vi "SubVI_ReadTDMs.vi"(8 "error in":errorcluster, 10 "Range Slide":cluster{dbl, dbl}={0.0, 1.0}, 11 "tdms文件输出":refnum<k34>) -> (0 "error out":errorcluster, 2 "WFM Out":waveform(dbl)[](array[waveform]), 3 "tdms file out":refnum<k34>)   [LabVIEW 2012]
panel:
  out "x*y":dbl
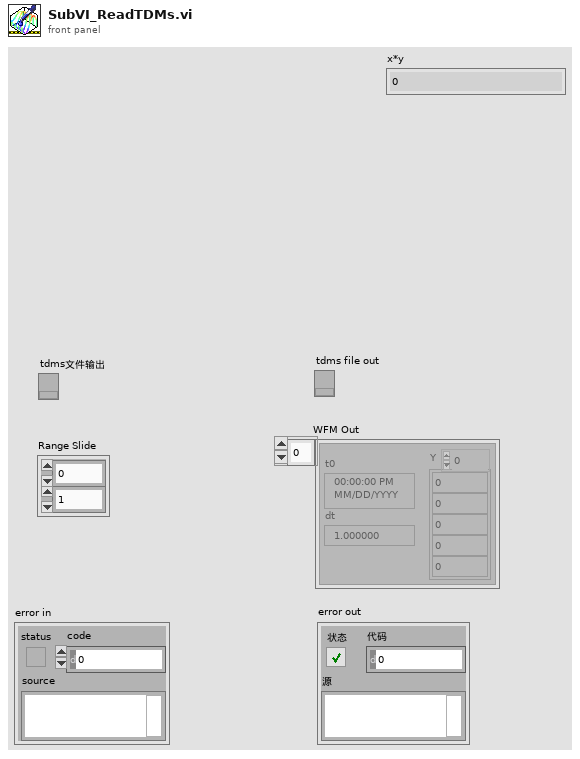
[diagram p1: front panel]
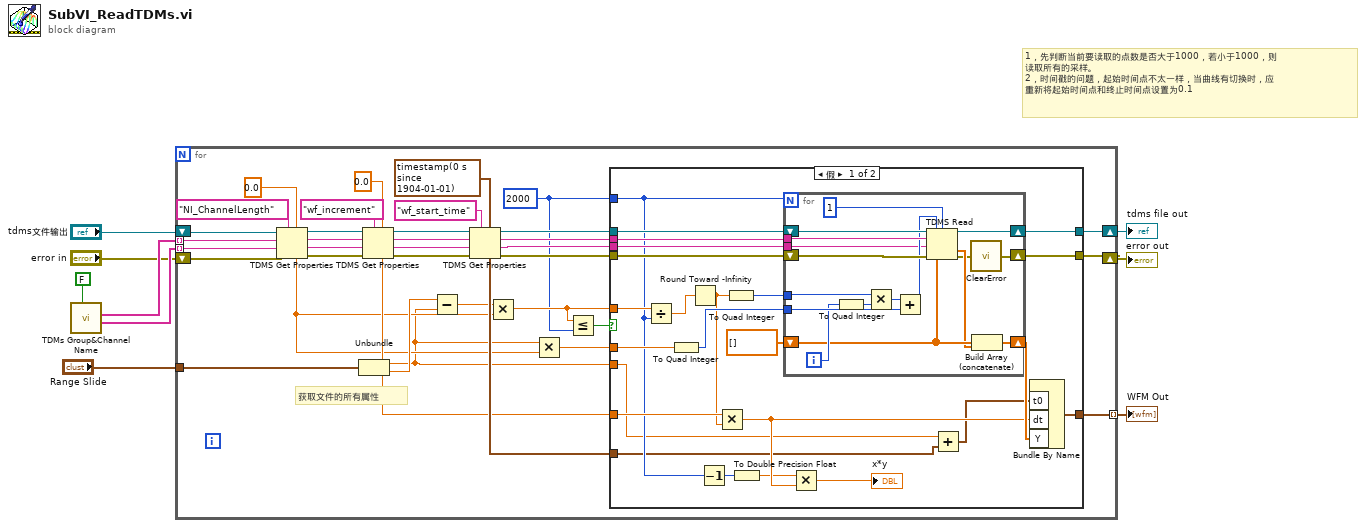
[diagram p0: block diagram]
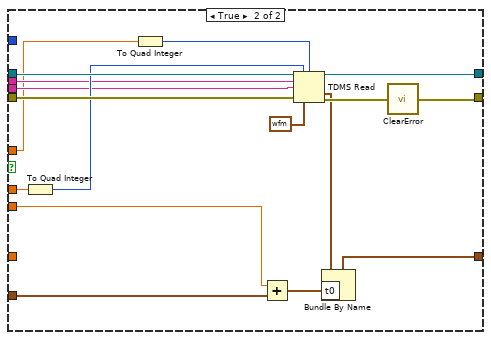
[diagram p2: hidden frame]
diagram:
  # "1，先判断当前要读取的点数是否大于1000，若小于1000，则\n读取所有的采样。\n2，时间戳的问题，起始时间点不太一样，当曲线有切换时，应\n重新将起始时间点和终止时间点设置为0.1"
  n1 = call "TDMs Group&Channel Name.vi"("Ini?"=FALSE) -> ("Channel"=w7:string[], "Group"=w8:string[])  [unwired: 8 in, 1 out]
  n2 = for {
    tunnel: [w44] -> w4 mode=indexing
    tunnel: w8 -> [w41] mode=indexing
    tunnel: w7 -> [w18] mode=indexing
    shift-right: [w15] -> w6
    shift-left: "tdms文件输出" -> [w43]
    shift-right: [w16] -> w5
    shift-left: "error in" -> [w42]
    tunnel: "Range Slide" -> [w14]
    w12 = 2000
    # "获取文件的所有属性"
    n3 = TDMS Get Properties(5:0.0, 7:"NI_ChannelLength", 8:w42, 9:w18, 10:w41, 11:w43) -> (0:w31:errorcluster, 1:w32:string, 2:w33:string, 3:w34:refnum<k34>, 4:w20:dbl)  [unwired: 1 out]
    n4 = Unbundle(w14) -> (w10:dbl, w38:dbl)
    n5 = TDMS Get Properties(5:0.0, 7:"wf_increment", 8:w31, 9:w32, 10:w33, 11:w34) -> (0:w27:errorcluster, 1:w22:string, 2:w25:string, 3:w29:refnum<k34>, 4:w21:dbl)  [unwired: 1 out]
    n6 = Subtract(x=w38, y=w10) -> (x-y=w19:dbl)
    n7 = TDMS Get Properties(5:timestamp(0 s since 1904-01-01), 7:"wf_start_time" ("属性名称"), 8:w27, 9:w22, 10:w25, 11:w29) -> (0:w26:errorcluster, 1:w17:string, 2:w24:string, 3:w28:refnum<k34>, 4:w45:timestamp)  [unwired: 1 out]
    n8 = Multiply(x=w19, y=w20) -> (x*y=w13:dbl)
    n9 = Multiply(x=w10, y=w20) -> (x*y=w37:dbl)
    n10 = Less Or Equal?(x=w13, y=w12) -> (x <= y?=w11:bool)
    n11 = case shown="假" w11 {
      tunnel: w45 -> [w48 w89]
      tunnel: [w67 w90] -> w44
      tunnel: w37 -> [w66 w101]
      tunnel: w28 -> [w63 w103]
      tunnel: w26 -> [w62 w102]
      tunnel: w24 -> [w61 w99]
      tunnel: w21 -> [w60 _]
      tunnel: w17 -> [w54 w98]
      tunnel: [w52 w94] -> w16
      tunnel: [w51 w96] -> w15
      tunnel: w13 -> [w50 w93]
      tunnel: w12 -> [w49 _]
      tunnel: w10 -> [w47 w88]
      frame False {
        n12 = Divide(x=w50, y=w49) -> (x/y=w64:dbl)
        n13 = To Quad Integer(1:w66) -> (0:w65:i64)
        n14 = Round Toward -Infinity(1:w64) -> (0:w56:dbl)
        n15 = Decrement(x=w49) -> (x-1=w58:i32)
        n16 = Multiply(x=w60, y=w56) -> (x*y=w68:dbl)
        n17 = To Quad Integer(1:w56) -> (0:w57:i64)
        n18 = To Double Precision Float(number=w58) -> (double precision float=w55:dbl)
        n19 = for {
          N: w49 -> [_]
          shift-right: [w83] -> w51
          shift-left: w63 -> [w86]
          shift-right: [w70] -> w52
          shift-left: w62 -> [w85]
          tunnel: w65 -> [w81]
          tunnel: w61 -> [w84]
          tunnel: w57 -> [w78]
          shift-right: [w76] -> w69
          shift-left: dbl[] [] -> [w75]
          tunnel: w54 -> [w73]
          i -> [w79]
          n20 = To Quad Integer(1:w79) -> (0:w74:i64)
          n21 = Multiply(x=w78, y=w74) -> (x*y=w77:i64)
          n22 = Add(x=w77, y=w81) -> (x+y=w80:i64)
          n23 = TDMS Read(0:w86, 1:w80, 2:1, 5:w84, 7:w73, 11:w85, 12:w75) -> (4:w83:refnum<k34>, 10:w72:dbl[], 15:w71:errorcluster)  [unwired: 1 in, 3 out]
          n24 = call <vilib>:"ClearError.vi"("error in (no error)"=w71) -> ("error out"=w70:errorcluster)
          n25 = Build Array (concatenate)(w75, w72) -> (w76:dbl[])
        }
        n26 = Multiply(x=w55, y=w68) -> (x*y=→"x*y":dbl)
        n27 = Add(x=w47, y=w48) -> (x+y=w46:timestamp)
        n28 = Bundle By Name("t0"=w46, "dt"=w68, "Y"=w69) -> (w67:waveform(dbl))  [unwired: 1 in]
      }
      frame True {
        n29 = To Quad Integer(1:w101) -> (0:w100:i64)
        n30 = To Quad Integer(1:w93) -> (0:w92:i64)
        n31 = Add(x=w88, y=w89) -> (x+y=w87:timestamp)
        n32 = TDMS Read(0:w103, 1:w100, 2:w92, 5:w99, 7:w98, 11:w102, 12:waveform(dbl) {"t0"=timestamp(0 s since 1904-01-01), "dt"=1.0, "Y"=[]} ("波形")) -> (4:w96:refnum<k34>, 10:w91:waveform(dbl), 15:w95:errorcluster)  [unwired: 1 in, 3 out]
        n33 = Bundle By Name(cluster=w91, "t0"=w87) -> (w90:waveform(dbl))
        n34 = call <vilib>:"ClearError.vi"("error in (no error)"=w95) -> ("error out"=w94:errorcluster)
      }
    }
  }
  "tdms file out" <- w6
  "error out" <- w5
  "WFM Out" <- w4
